vi "IntakeDeadband.vi"(10 "RightPwrIn":dbl, 11 "LeftPwrIn":dbl) -> (2 "RightPwrOut":dbl, 3 "LeftPwrOut":dbl)   [LabVIEW 2017]
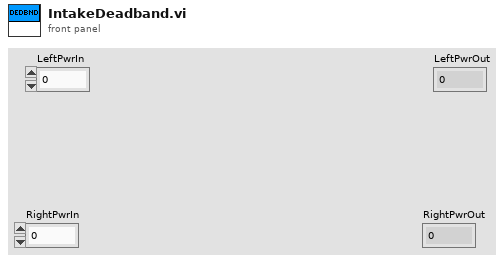
[diagram p1: front panel]
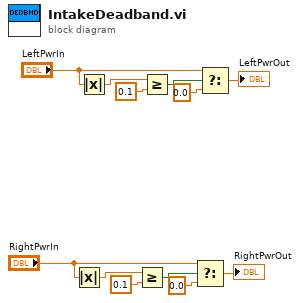
[diagram p0: block diagram]
diagram:
  n1 = Absolute Value(x="RightPwrIn") -> (abs(x)=w1:dbl)
  n2 = Absolute Value(x="LeftPwrIn") -> (abs(x)=w4:dbl)
  n3 = Greater Or Equal?(x=w1, y=0.1) -> (x >= y?=w5:bool)
  n4 = Greater Or Equal?(x=w4, y=0.1) -> (x >= y?=w12:bool)
  n5 = Select(t="RightPwrIn", s=w5, f=0.0) -> (s? t:f=→"RightPwrOut":dbl)
  n6 = Select(t="LeftPwrIn", s=w12, f=0.0) -> (s? t:f=→"LeftPwrOut":dbl)
